vi "uPublisher IsAlive.vi"(8 "error in (no error)":errorcluster, 11 "uClient_Publisher in":refnum<class "uClient_Publisher.lvclass">) -> (0 "error out":errorcluster, 2 "Is Alive?":bool, 3 "uClient_Publisher out":refnum<class "uClient_Publisher.lvclass">)   [LabVIEW 2021, in "uFramework.lvlib" / "uClient_Publisher.lvclass"]
uses:
  uClient_Publisher.lvclass
  U:/Projects/uFramework/Src/uFramework/uClient/uClient.lvclass
  uClient/uClient.lvclass/uClient.ctl
  uTransport/uTransport.lvclass
  uClient_Publisher.lvclass/uClient_Publisher.ctl
  uClient/uClient.lvclass
  U:/Projects/uFramework/Src/uFramework/uClient_Publisher/uClient_Publisher.lvclass
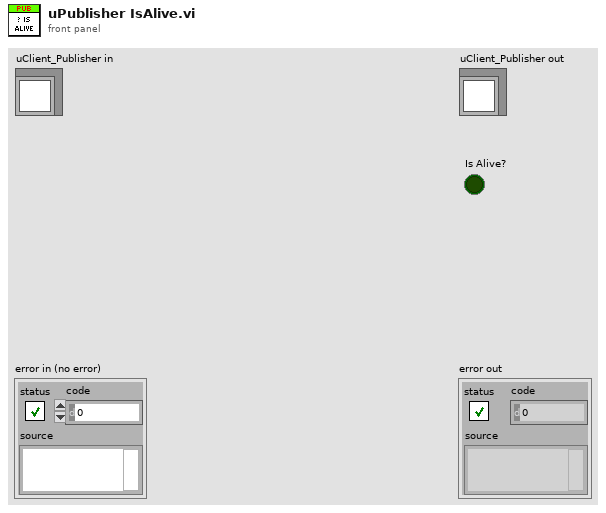
[diagram p1: front panel]
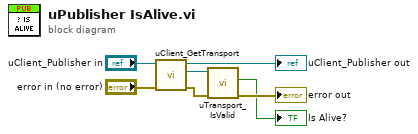
[diagram p0: block diagram]
diagram:
  n1 = call "uClient_GetTransport.vi"("error in (no error)"="error in (no error)", "uClient in"="uClient_Publisher in") -> ("error out"=w1:errorcluster, "uTransport"=w2:refnum<class "uTransport.lvclass">, "uClient out"=→"uClient_Publisher out":refnum<class "uClient_Publisher.lvclass">)  [unwired: 7 in]
  n2 = call-dynamic "uTransport_IsValid.vi"("error in (no error)"=w1, "uTransport in"=w2) -> ("error out"=→"error out":errorcluster, "IsValid?"=→"Is Alive?":bool)  [unwired: 7 in, 1 out]
